vi "CRCTester.vi"() -> ()   [LabVIEW 2016]
uses:
  Common_FPGA_Modbus/DataTypes/ModbusCRC32Settings.ctl
  <vilib>/rvi/DataTransferAndStorage/Container/Common/niFpgaContainerExecOnDevCompGetState.vi
  <vilib>/rvi/Emulation/niFpgaEmulationIsFPGAContextNoSignature.vi
  <vilib>/rvi/Emulation/niFpgaSctlEmulationGetInTimedLoop.vi
  <vilib>/rvi/errors/niFpgaSetErrorForExecOnDevCompSimple.vi
  <vilib>/rvi/eio/common/nirviEmuReportErrorAndStop.vi
  <vilib>/rvi/DataTransferAndStorage/Container/Common/niFpgaContainerGetUniqueNameForEmu.vi
  <vilib>/rvi/FIFO/Fifo_Resource/nirvififoEmulationSetSize.vi
  <vilib>/rvi/FIFO/Fifo_Resource/nirviFifoEmulationQueueMgr.vi
  <instcachedir>/0/nirviFifoEmulationQueueMgr_E5CAEC123FF24DC58D834DCA3CDAA9B5.lvgen/nirviFifoEmulationQueueMgr_E5CAEC123FF24DC58D834DCA3CDAA9B5_000.vi
  <vilib>/rvi/FIFO/Fifo_Resource/nirvififoEmulationDetermineInputValidOut.vi
  <vilib>/rvi/FIFO/Fifo_Resource/nirvififoEmulationCreateLock.vi
  <vilib>/rvi/Emulation/niFpgaProcessEmulError.vi
  <vilib>/rvi/FIFO/Fifo_Resource/nirvififoEmulationObtainLock.vi
  <vilib>/rvi/FIFO/Fifo_Resource/nirvififoEmulationReleaseLock.vi
  <vilib>/rvi/occurrence/nirviWaitOnOccurrenceBase.vi
  <vilib>/rvi/errors/nirviReportUnexpectedCaseInternalError.vi
  <vilib>/rvi/errors/nirviReportUnexpectedCaseInternalError (U32).vi
  <vilib>/Utility/error.llb/Clear Errors.vi
  <vilib>/rvi/interface/RandomDataEmulation/niFpgaRandomDataHandleErrors.vi
  <instcachedir>/0/nirviFifoEmulationQueueMgr_E5CAEC123FF24DC58D834DCA3CDAA9B5.lvgen/nirviFifoEmulationQueueMgr_E5CAEC123FF24DC58D834DCA3CDAA9B5_001.vi
  <vilib>/rvi/DataTransferAndStorage/Container/XNode/niFpgaContainer.xnode
  <vilib>/rvi/FIFO/Fifo_Resource/niFpgaFifoEmulationRefIn.vi
  Common_FPGA_Modbus/FPGAModbus.lvlib
panel:
  out "CRCStream":u8[](array[numeric])
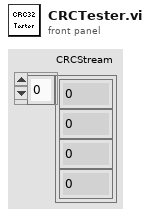
[diagram p1: front panel]
types:
  T1 = typedef "FPGAModbus.lvlib/ModbusCRC32Settings.ctl" = cluster{"DataFIFO":refnum<k21>, "CalculateFIFO":refnum<k21>, "OutputFIFO":refnum<k21>}
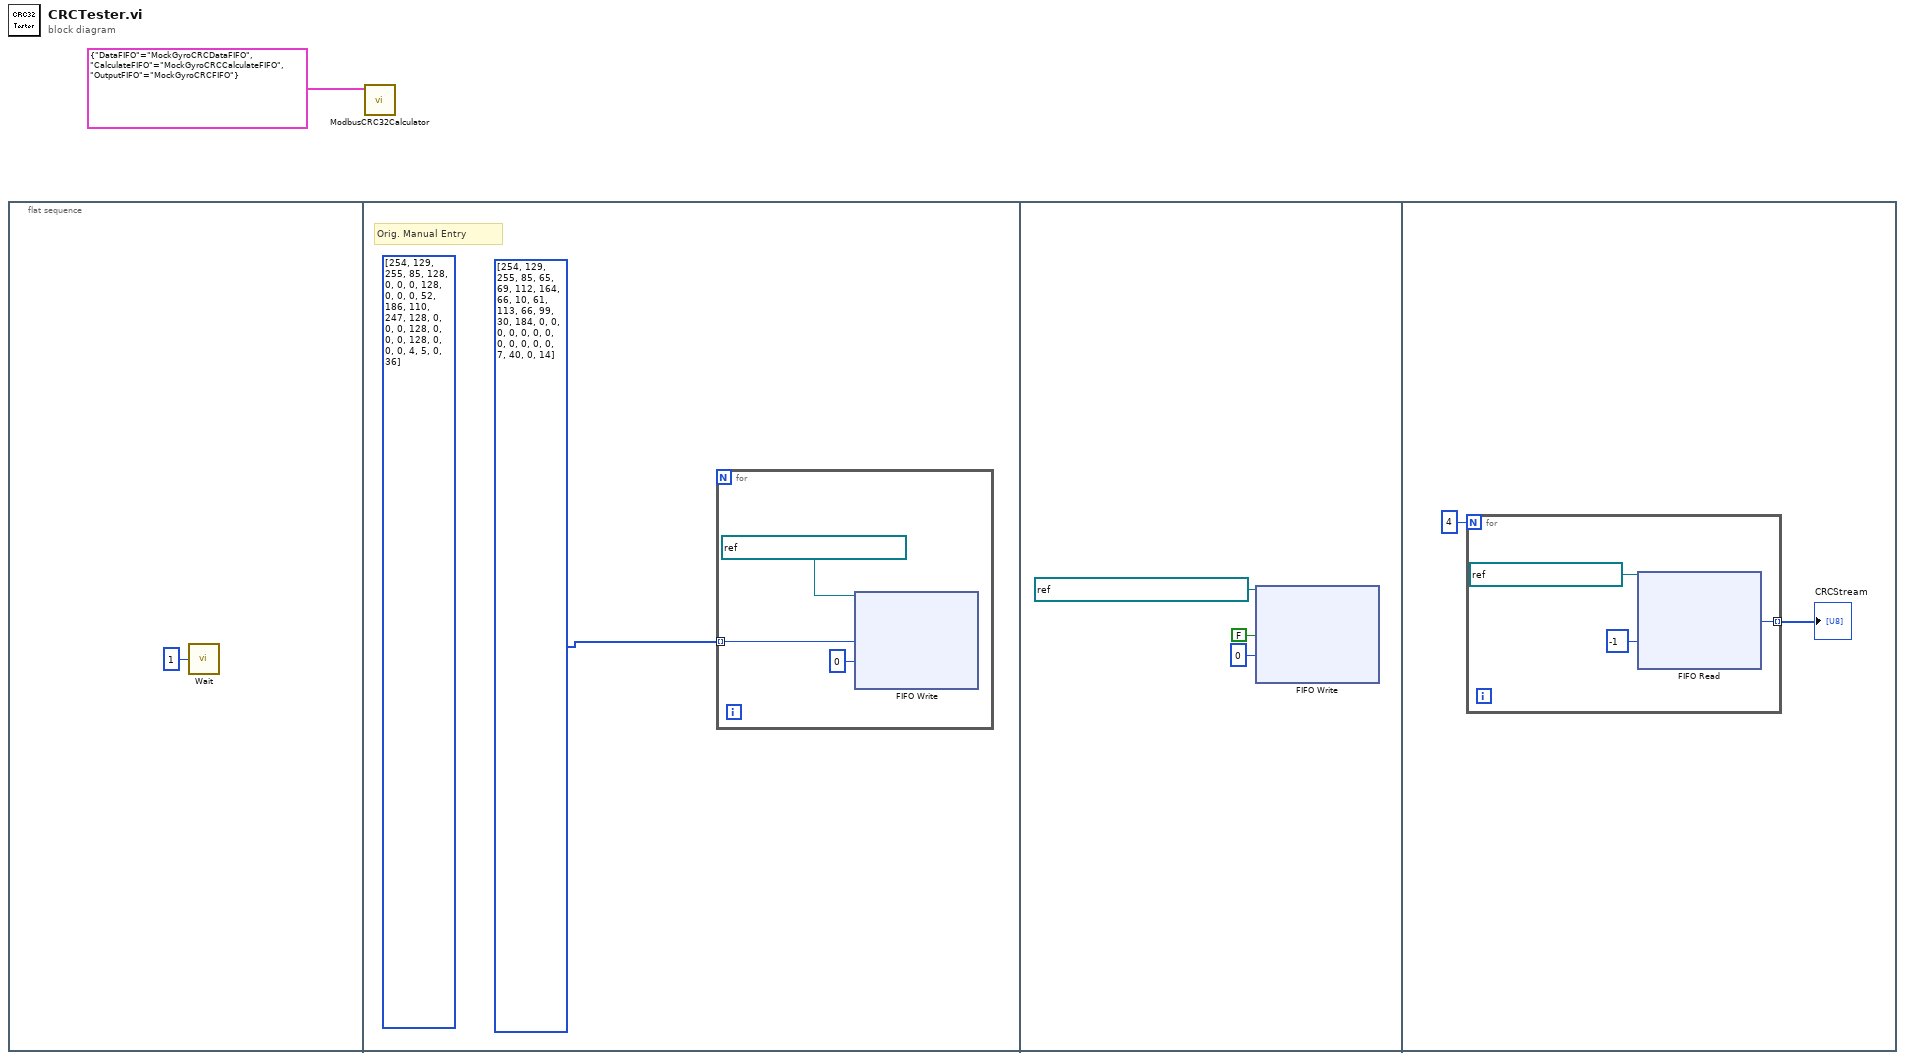
[diagram p0: block diagram]
diagram:
  n1 = flat-sequence {
    frame #0 {
      n2 = call "Wait"("Count(mSec)"=u32 1) -> ()  [unwired: 1 out]
    }
    frame #1 {
      (unwired) u8[] [254, 129, 255, 85, 128, 0, 0, 0, 128, 0, 0, 0, 52, 186, 110, 247, 128, 0, 0, 0, 128, 0, 0, 0, 128, 0, 0, 0, 4, 5, 0, 36]
      # "Orig. Manual Entry"
      n3 = for {
        tunnel: u8[] [254, 129, 255, 85, 65, 69, 112, 164, 66, 10, 61, 113, 66, 99, 30, 184, 0, 0, 0, 0, 0, 0, 0, 0, 0, 0, 0, 0, 7, 40, 0, 14] -> [w5] mode=indexing
        n4 = xnode ("FIFO Write")("Element"=w5, "Timeout"=0, "FIFO In"=refnum<k21> "MockGyroCRCDataFIFO" ("DataFIFO")) -> ()  [unwired: 2 out]
      }
    }
    frame #2 {
      n5 = xnode ("FIFO Write")("Element"=FALSE, "Timeout"=0, "FIFO In"=refnum<k21> "MockGyroCRCCalculateFIFO" ("CalculateFIFO")) -> ()  [unwired: 2 out]
    }
    frame #3 {
      n6 = for {
        N: 4 -> [_]
        tunnel: [w12] -> w10 mode=indexing
        n7 = xnode ("FIFO Read")("Timeout"=-1, "FIFO In"=refnum<k21> "MockGyroCRCFIFO" ("OutputFIFO")) -> ("Element"=w12:u8)  [unwired: 2 out]
      }
      "CRCStream" <- w10
    }
  }
  n8 = call "ModbusCRC32Calculator.vi"("ModbusCRC32Settings"=T1 {"DataFIFO"="MockGyroCRCDataFIFO", "CalculateFIFO"="MockGyroCRCCalculateFIFO", "OutputFIFO"="MockGyroCRCFIFO"}) -> ()  [unwired: 11 in]
